vi "Sort Local and Target Virt Instrs.vi"(8 "error in":errorcluster, 11 "Virt Instr CFGs":T1(array[cluster])) -> (0 "error out":errorcluster, 2 "Local Virt Instrs":T2(array[cluster]), 3 "Target Virt Instrs":T1(array[cluster]))   [LabVIEW 2024, in "HAL.lvlib" / "MSS.lvclass"]
uses:
  MSS.lvclass
  Virtual Instruments/Perform Action Remote Strategy.lvclass
  adeec9ff-388a-446b-91ea-ac47482ef736.vi
  adeec9ff-388a-446b-91ea-ac47482ef736.vi/a4169a97-72fc-4003-a778-603cf20cafa0.vi
  <vilib>/JDP Science/JSONtext/Find Item.vi
  <vilib>/JDP Science/JSONtext/Next JSON Value.vi
  <vilib>/JDP Science/JSONtext/String Subset.vi
  <vilib>/JDP Science/JSONtext/Parsing/Advance past next JSON Value (inlined COPY).vi
  <vilib>/JDP Science/JSONtext/Parsing/Advance past whitespace.vi
  <vilib>/JDP Science/JSONtext/Parsing/Advance past String.vi
  <vilib>/JDP Science/JSONtext/Parsing/Advance past Number.vi
  <vilib>/JDP Science/JSONtext/Parsing/Advance past Line Ending.vi
  <vilib>/JDP Science/JSONtext/Parsing/Parse Full Path or Item Name.vi
  <vilib>/JDP Science/JSONtext/Parsing/Advance past Array.vi
  <vilib>/JDP Science/JSONtext/Parsing/Advance past Object.vi
  <vilib>/JDP Science/JSONtext/support/Error Cluster From Code.vi
  <vilib>/JDP Science/JSONtext/Offset/Find Item Locations by Path.vi
  <vilib>/JDP Science/JSONtext/JSON text to Variant.vi
  <vilib>/Utility/error.llb/Error Cluster From Error Code.vi
  <vilib>/JDP Science/JSONtext/LVClass Serializer/JSONtext LVClass Serializer.lvclass
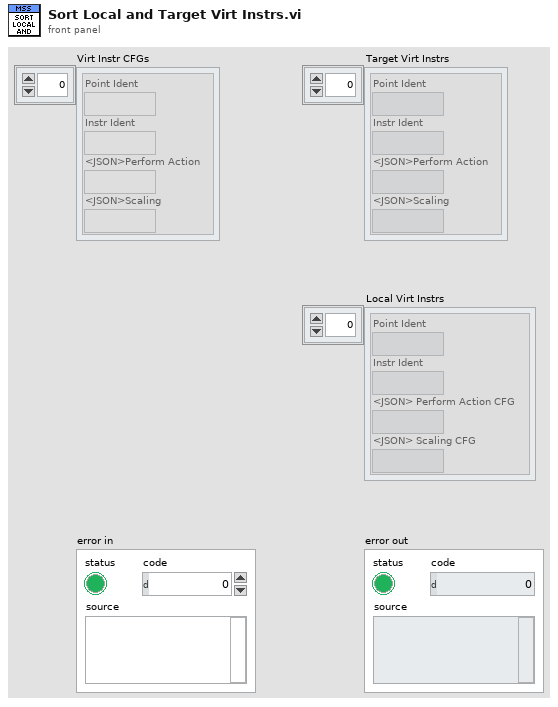
[diagram p1: front panel]
types:
  T1 = cluster{"Point Ident":string, "Instr Ident":string, "<JSON>Perform Action":string, "<JSON>Scaling":string}[]
  T2 = cluster{"Point Ident":string, "Instr Ident":string, "<JSON> Perform Action CFG":string, "<JSON> Scaling CFG":string}[]
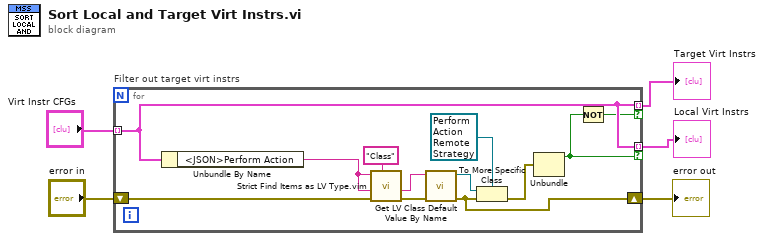
[diagram p0: block diagram]
diagram:
  n1 = for "Filter out target virt instrs" {
    tunnel: "Virt Instr CFGs" -> [w8] mode=indexing
    shift-right: [w11] -> w4
    shift-left: "error in" -> [w12]
    tunnel: [w8] -> w3 mode=indexing if=w7
    tunnel: [w8] -> w2 mode=indexing if=w9
    n2 = Unbundle By Name(w8) -> ("<JSON>Perform Action"=w6:string)
    n3 = call "Strict Find Items as LV Type.vim"("$Path or Item Name"="Class", "error in"=w12, "Data Type and Default Value"=w6, "<JSON>"=w6) -> ("error out"=w16:errorcluster, "Data out"=w13:string)  [unwired: 5 in, 1 out]
    n4 = call <vilib>:"Get LV Class Default Value By Name.vi"("error in (no error)"=w16, "class name"=w13) -> ("error out"=w11:errorcluster, "object"=w14:refnum<class>)  [unwired: 8 in]
    n5 = To More Specific Class(target class=refnum<class "Perform Action Remote Strategy.lvclass"> refnum ("HAL.lvlib:Remote Action Performance.lvclass"), reference=w14, error in=w11) -> (error out=w10:errorcluster)  [unwired: 1 out]
    n6 = Unbundle(w10) -> ("status"=w9:bool)  [unwired: 2 out]
    n7 = Not(x=w9) -> (.not. x?=w7:bool)
  }
  "error out" <- w4
  "Local Virt Instrs" <- w2
  "Target Virt Instrs" <- w3
